vi "Main_Module.vi"(0 "A":dbl, 5 "B":dbl, 11 "Error_In":errorcluster) -> (4 "C":dbl, 15 "Error_Out":errorcluster)   [LabVIEW 2023]
doc: "This is the Main Module that perform the calculator."
uses:
  Controls/Calculator_Operation_Select.ctl
  Controls/Queue_Operation_Select.ctl
  Controls/Calculator_Data.ctl
  Classes/Calculator/Calculator.lvclass
  Controls/State_and_Data.ctl
  Classes/Calculator/Children/Multiplication/Multiplication.lvclass
  D:/Git/Assignments/Assignment-24/Assignment-24_LV23V/Classes/Calculator/Calculator.lvclass
  Classes/Calculator/Children/Division/Division.lvclass
  Classes/Calculator/Children/Addition/Addition.lvclass
  Classes/Calculator/Children/Subtraction/Subtraction.lvclass
panel:
  in  "Operation":T1
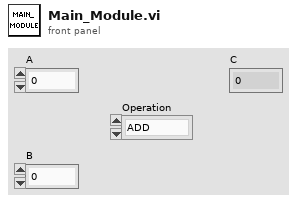
[diagram p1: front panel]
types:
  T1 = typedef "Calculator_Operation_Select.ctl" = enum16{"ADD", "SUB", "MUL", "DIV"}
  T2 = typedef "State_and_Data.ctl" = cluster{"State":string, "Data":variant}
  T3 = typedef "Queue_Operation_Select.ctl" = enum16{"Obtain_Queue", "Enqueue", "Enqueue_First", "Enqueue_N", "Lossy_Enqueue", "Preview", "Queue_Status", "Dequeue", "Flush", "Release_Queue"}
  T4 = typedef "Calculator_Data.ctl" = cluster{"Inputs":dbl[], "Operation":T1, "Parent_Calculator":refnum<class "Calculator.lvclass">[], "C":dbl, "State_and_Data":T2}
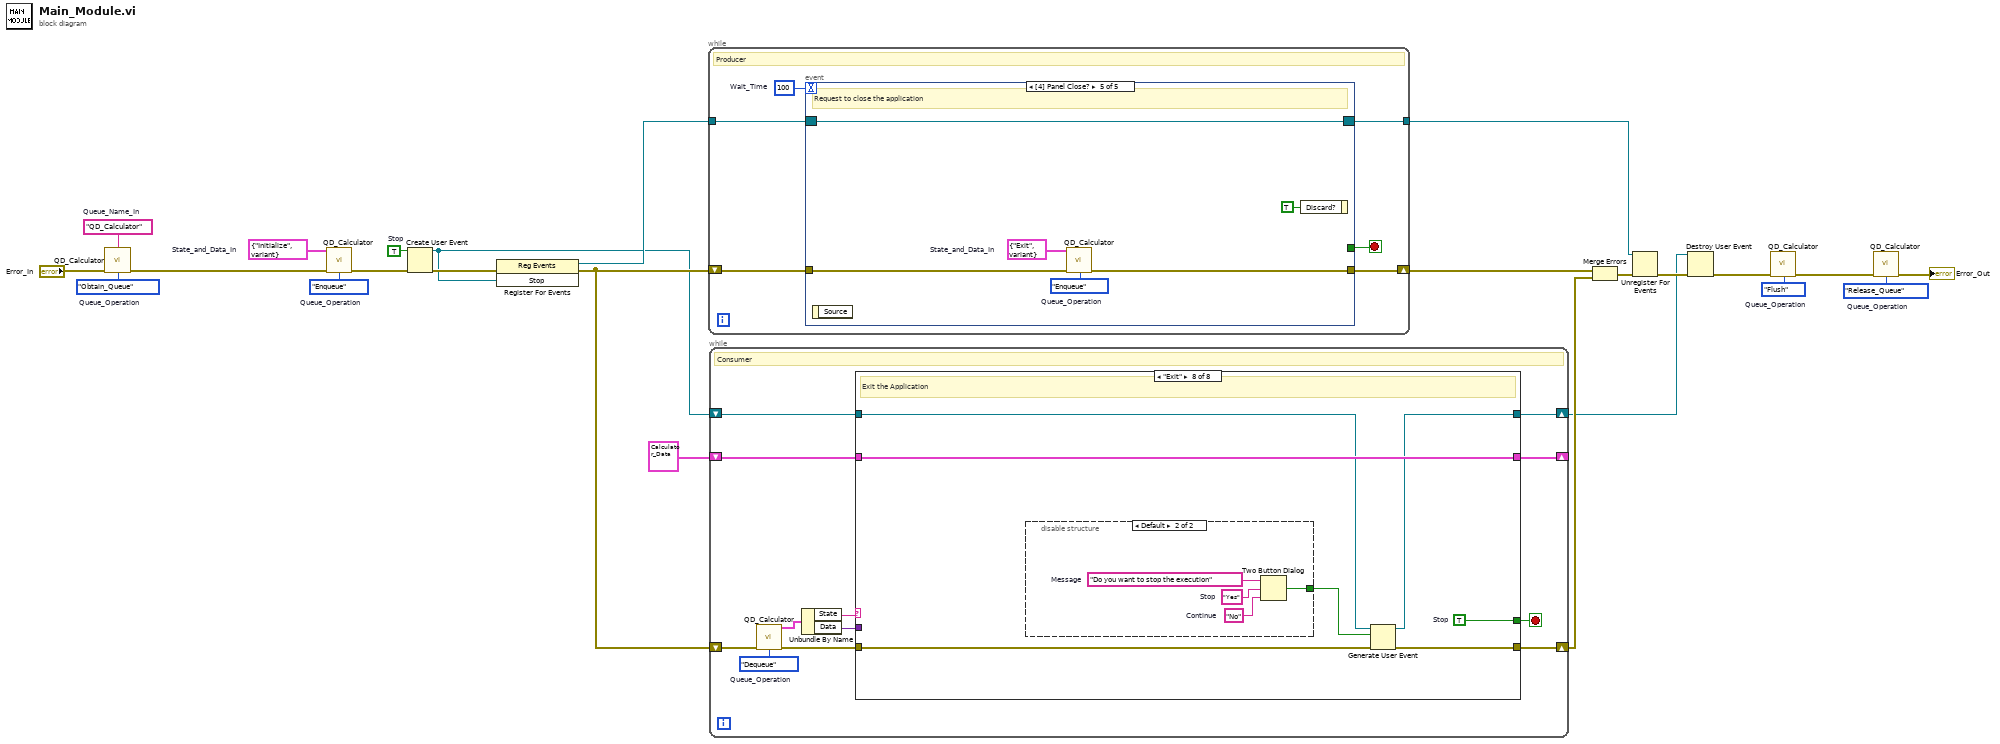
[diagram p0: block diagram]
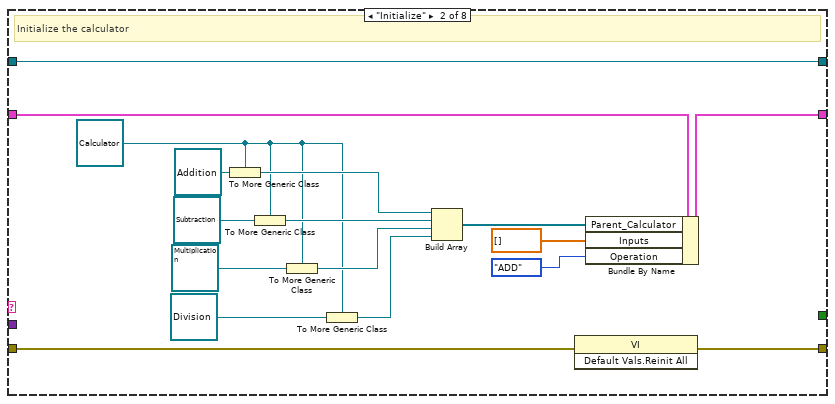
[diagram p3: hidden frame]
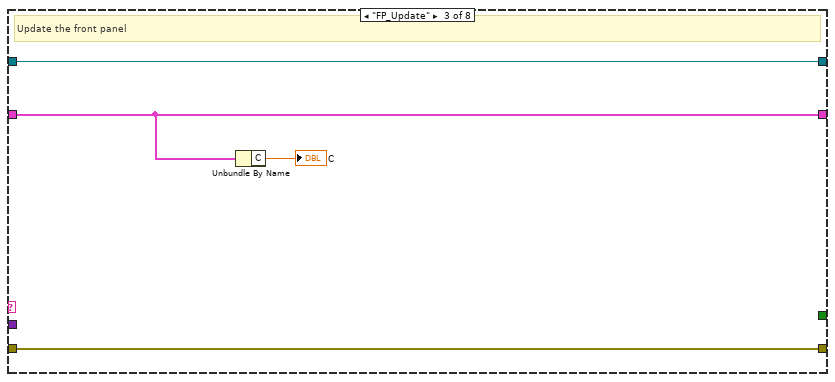
[diagram p4: hidden frame]
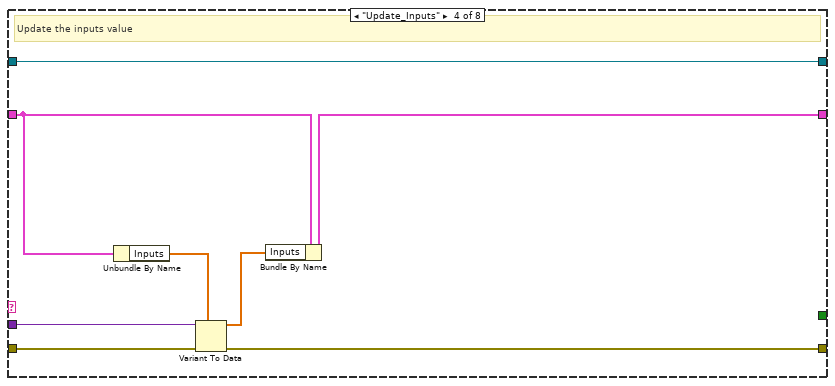
[diagram p5: hidden frame]
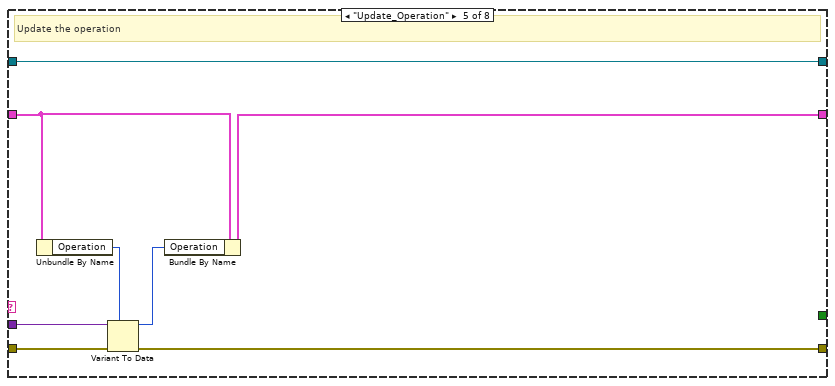
[diagram p6: hidden frame]
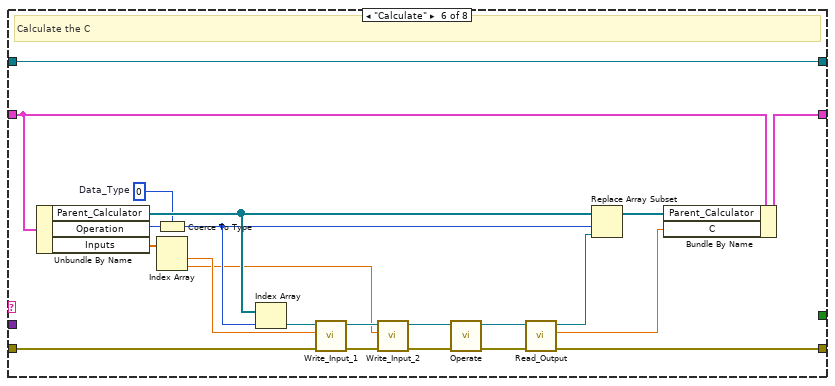
[diagram p7: hidden frame]
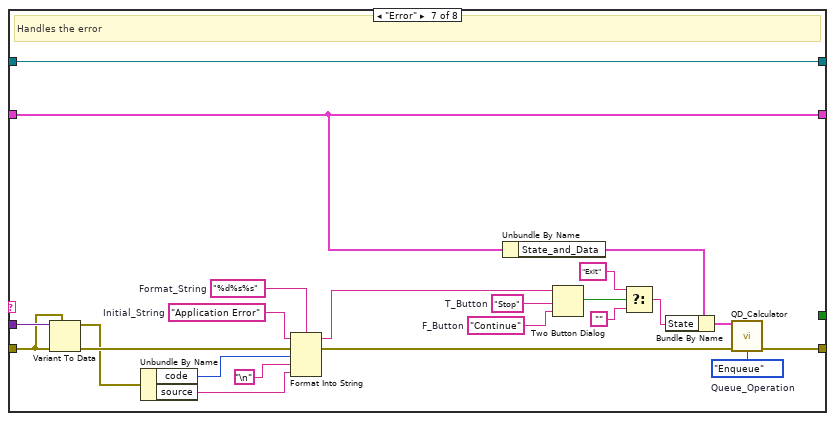
[diagram p8: hidden frame]
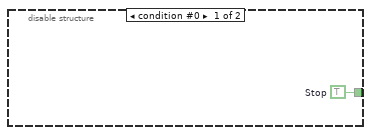
[diagram p9: hidden frame]
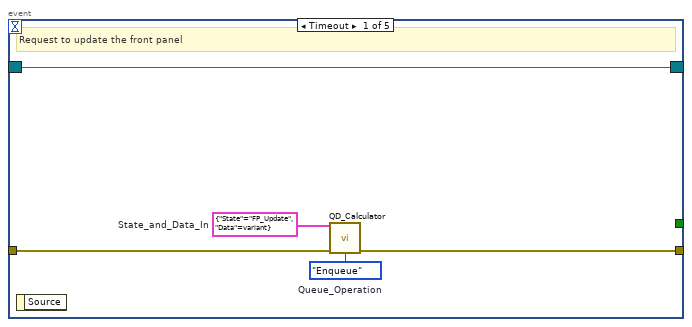
[diagram p10: hidden frame]
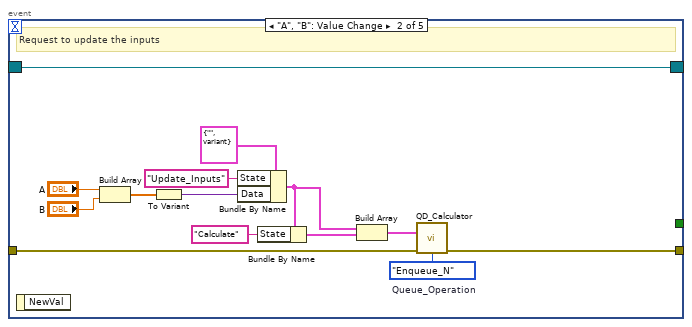
[diagram p11: hidden frame]
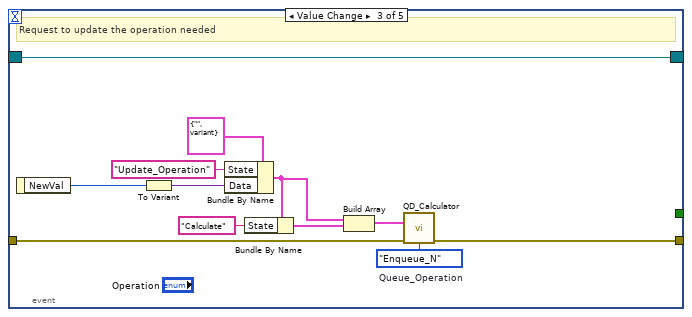
[diagram p12: hidden frame]
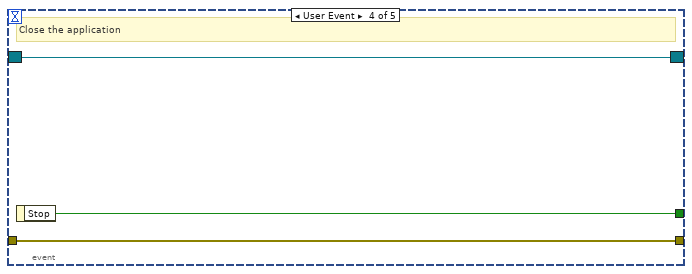
[diagram p13: hidden frame]
diagram:
  w1 = T2 {"State"="Initialize", "Data"=variant}  # State_and_Data_In
  w2 = Queue_Operation_Select."Release_Queue"  # Queue_Operation
  w3 = Queue_Operation_Select."Flush"  # Queue_Operation
  w6 = TRUE  # Stop
  w16 = "QD_Calculator"  # Queue_Name_In
  w17 = Queue_Operation_Select."Enqueue"  # Queue_Operation
  w18 = Queue_Operation_Select."Obtain_Queue"  # Queue_Operation
  n1 = call "QD_Calculator.vi"("Queue_Name_In"=w16, "Error_In"="Error_In", "Queue_Operation"=w18) -> ("Error_Out"=w20:errorcluster)  [unwired: 10 in, 2 out]
  n2 = call "QD_Calculator.vi"("State_and_Data_In"=w1, "Error_In"=w20, "Queue_Operation"=w17) -> ("Error_Out"=w19:errorcluster)  [unwired: 10 in, 2 out]
  n3 = Create User Event(user event datatype=w6, error in=w19) -> (user event=w7:refnum<user-event>, error out=w14:errorcluster)
  n4 = register-events(error in=w14, w7) -> (reference out=w12:refnum<event-registration>, error out=w13:errorcluster)  [unwired: 1 in]
  n5 = while {
    shift-right: [w29] -> w24
    shift-left: w13 -> [w30]
    tunnel: w12 -> [w27]
    tunnel: [w26] -> w10
    stop <- w25 stop-if-true
    w28 = 100  # Wait_Time
    # "Producer"
    n6 = event shown="[4] Panel Close?" {
      selector: w27 -> [w34 w39 w50 w62 w65]
      dyn-events: [w34 w39 w50 w62 w65] -> w26
      timeout: w28 -> [_ _ _ _ _]
      tunnel: w30 -> [w35 w40 w61 w64 w70]
      tunnel: [w33 w41 w60 w64 w69] -> w29
      tunnel: [_ _ _ w63 _] -> w25
      event Timeout {
        w31 = T2 {"State"="FP_Update", "Data"=variant}  # State_and_Data_In
        w32 = Queue_Operation_Select."Enqueue"  # Queue_Operation
        # "Request to update the front panel"
        n7 = event-data() -> ()  [unwired: 1 in, 1 out]
        n8 = call "QD_Calculator.vi"("State_and_Data_In"=w31, "Error_In"=w35, "Queue_Operation"=w32) -> ("Error_Out"=w33:errorcluster)  [unwired: 10 in, 2 out]
      }
      event "A", "B": Value Change {
        w49 = Queue_Operation_Select."Enqueue_N"  # Queue_Operation
        # "Request to update the inputs"
        n9 = event-data() -> ()  [unwired: 1 in, 1 out]
        n10 = Build Array("A", "B") -> (w36:dbl[])
        n11 = To Variant(anything=w36) -> (Variant=w47:variant)
        n12 = Bundle By Name(cluster=T2 {"State"="", "Data"=variant} ("State_and_Data"), "State"="Update_Inputs", "Data"=w47) -> (w45:T2)
        n13 = Bundle By Name(cluster=w45, "State"="Calculate") -> (w44:T2)
        n14 = Build Array(w45, w44) -> (w43:T2[])
        n15 = call "QD_Calculator.vi"("State_and_Data_N_In"=w43, "Error_In"=w40, "Queue_Operation"=w49) -> ("Error_Out"=w41:errorcluster)  [unwired: 10 in, 2 out]
      }
      event Value Change {
        w59 = Queue_Operation_Select."Enqueue_N"  # Queue_Operation
        # "Request to update the operation needed"
        n16 = event-data() -> ("NewVal"=w57:T1)  [unwired: 1 in]
        n17 = To Variant(anything=w57) -> (Variant=w56:variant)
        n18 = Bundle By Name(cluster=T2 {"State"="", "Data"=variant} ("State_and_Data"), "State"="Update_Operation", "Data"=w56) -> (w54:T2)
        n19 = Bundle By Name(cluster=w54, "State"="Calculate") -> (w53:T2)
        n20 = Build Array(w54, w53) -> (w52:T2[])
        n21 = call "QD_Calculator.vi"("State_and_Data_N_In"=w52, "Error_In"=w61, "Queue_Operation"=w59) -> ("Error_Out"=w60:errorcluster)  [unwired: 10 in, 2 out]
      }
      event User Event {
        # "Close the application"
        n22 = event-data() -> ("Stop"=w63:bool)  [unwired: 1 in]
      }
      event Panel Close? {
        w67 = T2 {"State"="Exit", "Data"=variant}  # State_and_Data_In
        w68 = Queue_Operation_Select."Enqueue"  # Queue_Operation
        # "Request to close the application"
        n23 = event-data() -> ()  [unwired: 1 in, 1 out]
        n24 = call "QD_Calculator.vi"("State_and_Data_In"=w67, "Error_In"=w70, "Queue_Operation"=w68) -> ("Error_Out"=w69:errorcluster)  [unwired: 10 in, 2 out]
        n25 = event-data("Discard?"=TRUE) -> ()  [unwired: 1 in, 1 out]
      }
    }
  }
  n26 = while {
    shift-right: [w81] -> w21
    shift-left: w13 -> [w82]
    shift-right: [w75] -> _
    shift-left: T4 {"Inputs"=[], "Operation"=enum."ADD", "Parent_Calculator"=[], "C"=0.0, "State_and_Data"={"State"="", "Data"=variant}} -> [w74]
    shift-right: [w73] -> w8
    shift-left: w7 -> [w72]
    stop <- w71 stop-if-true
    w79 = Queue_Operation_Select."Dequeue"  # Queue_Operation
    # "Consumer"
    n27 = call "QD_Calculator.vi"("Error_In"=w82, "Queue_Operation"=w79) -> ("State_and_Data_Out"=w78:T2, "Error_Out"=w80:errorcluster)  [unwired: 11 in, 1 out]
    n28 = Unbundle By Name(w78) -> ("State"=w77:string, "Data"=w76:variant)
    n29 = case shown="\"Exit\"" w77 {
      tunnel: w80 -> [w85 w102 w106 w114 w122 w143 w150 w174]
      tunnel: [w85 w86 w106 w113 w121 w135 w147 w172] -> w81
      tunnel: w76 -> [_ _ _ w112 w120 _ w151 _]
      tunnel: [w84 w100 w104 w109 w117 w137 w153 w173] -> w75
      tunnel: w74 -> [w84 w101 w104 w110 w118 w144 w153 w173]
      tunnel: [w83 w87 w105 w107 w115 w127 w167 w170] -> w73
      tunnel: w72 -> [w83 w87 w105 w107 w115 w127 w167 w171]
      tunnel: [_ _ _ _ _ _ _ w169] -> w71
      frame Default {
      }
      frame "Initialize" {
        w90 = refnum<class "Calculator.lvclass"> refnum ("Calculator.lvclass")
        # "Initialize the calculator"
        n30 = To More Generic Class(target class=w90, reference=refnum<class "Addition.lvclass"> refnum ("Addition.lvclass")) -> (generic class reference=w94:refnum<class "Calculator.lvclass">)
        n31 = To More Generic Class(target class=w90, reference=refnum<class "Subtraction.lvclass"> refnum ("Subtraction.lvclass")) -> (generic class reference=w93:refnum<class "Calculator.lvclass">)
        n32 = To More Generic Class(target class=w90, reference=refnum<class "Multiplication.lvclass"> refnum ("Multiplication.lvclass")) -> (generic class reference=w92:refnum<class "Calculator.lvclass">)
        n33 = To More Generic Class(target class=w90, reference=refnum<class "Division.lvclass"> refnum ("Division.lvclass")) -> (generic class reference=w91:refnum<class "Calculator.lvclass">)
        n34 = Build Array(w94, w93, w92, w91) -> (w95:refnum<class "Calculator.lvclass">[])
        n35 = invoke class="VI" method="Default Vals.Reinit All"(error in=w102) -> (error out=w86:errorcluster)  [unwired: 2 in, 2 out]
        n36 = Bundle By Name(cluster=w101, "Parent_Calculator"=w95, "Inputs"=dbl[] [] ("A"), "Operation"=Calculator_Operation_Select."ADD") -> (w100:T4)
      }
      frame "FP_Update" {
        # "Update the front panel"
        n37 = Unbundle By Name(w104) -> ("C"=→"C":dbl)
      }
      frame "Update_Inputs" {
        # "Update the inputs value"
        n38 = Unbundle By Name(w110) -> ("Inputs"=w111:dbl[])
        n39 = Variant To Data(error in=w114, type=w111, Variant=w112) -> (data=w108:dbl[], error out=w113:errorcluster)
        n40 = Bundle By Name(cluster=w110, "Inputs"=w108) -> (w109:T4)
      }
      frame "Update_Operation" {
        # "Update the operation"
        n41 = Unbundle By Name(w118) -> ("Operation"=w119:T1)
        n42 = Variant To Data(error in=w122, type=w119, Variant=w120) -> (data=w116:T1, error out=w121:errorcluster)
        n43 = Bundle By Name(cluster=w118, "Operation"=w116) -> (w117:T4)
      }
      frame "Calculate" {
        w128 = 0  # Data_Type
        # "Calculate the C"
        n44 = Unbundle By Name(w144) -> ("Parent_Calculator"=w133:refnum<class "Calculator.lvclass">[], "Operation"=w132:T1, "Inputs"=w125:dbl[])
        n45 = Coerce To Type(0:w132, 1:w128) -> (2:w129:i32)
        n46 = Index Array(array=w125) -> (element #1=w124:dbl, element #2=w123:dbl)  [unwired: 2 in]
        n47 = Index Array(array=w133, index=w129) -> (element=w140:refnum<class "Calculator.lvclass">)
        n48 = call-dynamic "Write_Input_1.vi"("Error_In"=w143, "Input_1"=w124, "Calculator_In"=w140) -> ("Error_Out"=w142:errorcluster, "Calculator_Out"=w126:refnum<class "Calculator.lvclass">)  [unwired: 7 in]
        n49 = call-dynamic "Write_Input_2.vi"("Error_In"=w142, "Input_2"=w123, "Calculator_In"=w126) -> ("Error_Out"=w141:errorcluster, "Calculator_Out"=w139:refnum<class "Calculator.lvclass">)  [unwired: 7 in]
        n50 = call-dynamic "Operate.vi"("Error_In"=w141, "Calculator_In"=w139) -> ("Error_Out"=w136:errorcluster, "Calculator_Out"=w138:refnum<class "Calculator.lvclass">)  [unwired: 8 in]
        n51 = call-dynamic "Read_Output.vi"("Error_In"=w136, "Calculator_In"=w138) -> ("Error_Out"=w135:errorcluster, "Output"=w130:dbl, "Calculator_Out"=w131:refnum<class "Calculator.lvclass">)  [unwired: 7 in]
        n52 = Replace Array Subset(array=w133, new element=w131, index=w129) -> (w134:refnum<class "Calculator.lvclass">[])
        n53 = Bundle By Name(cluster=w144, "Parent_Calculator"=w134, "C"=w130) -> (w137:T4)
      }
      frame "Error" {
        w145 = Queue_Operation_Select."Enqueue"  # Queue_Operation
        w162 = "%d%s%s"  # Format_String
        w163 = "Application Error"  # Initial_String
        w164 = "Stop"  # T_Button
        w165 = "Continue"  # F_Button
        # "Handles the error"
        n54 = Variant To Data(error in=w150, type=w150, Variant=w151) -> (data=w149:errorcluster, error out=w152:errorcluster)
        n55 = Unbundle By Name(w149) -> ("code"=w160:i32, "source"=w159:string)
        n56 = Format Into String(format string=w162, initial string=w163, error in=w152, w160, "\n", w159) -> (resulting string=w166:string, error out=w154:errorcluster)
        n57 = Unbundle By Name(w153) -> ("State_and_Data"=w148:T2)
        n58 = Two Button Dialog(message=w166, 1:w165, 2:w164) -> (T button?=w157:bool)
        n59 = Select(t="Exit" ("State"), s=w157, f="") -> (s? t:f=w155:string)
        n60 = Bundle By Name(cluster=w148, "State"=w155) -> (w146:T2)
        n61 = call "QD_Calculator.vi"("State_and_Data_In"=w146, "Error_In"=w154, "Queue_Operation"=w145) -> ("Error_Out"=w147:errorcluster)  [unwired: 10 in, 2 out]
      }
      frame "Exit" {
        w169 = TRUE  # Stop
        # "Exit the Application"
        n62 = disable-structure shown="Default" {
          disable-tunnel: [w175 w176] -> w168
          frame condition #0 {
            w175 = TRUE  # Stop
          }
          frame condition #1 (active) {
            w177 = "No"  # Continue
            w178 = "Yes"  # Stop
            w179 = "Do you want to stop the execution"  # Message
            n63 = Two Button Dialog(message=w179, 1:w177, 2:w178) -> (T button?=w176:bool)
          }
        }
        n64 = Generate User Event(user event=w171, event data cluster=w168, error in=w174) -> (user event out=w170:refnum<user-event>, error out=w172:errorcluster)  [unwired: 1 in]
      }
    }
  }
  n65 = Merge Errors(w24, w21) -> (w22:errorcluster)
  n66 = Unregister For Events(event registration refnum=w10, error in=w22) -> (error out=w11:errorcluster)
  n67 = Destroy User Event(user event=w8, error in=w11) -> (error out=w9:errorcluster)
  n68 = call "QD_Calculator.vi"("Error_In"=w9, "Queue_Operation"=w3) -> ("Error_Out"=w4:errorcluster)  [unwired: 11 in, 2 out]
  n69 = call "QD_Calculator.vi"("Error_In"=w4, "Queue_Operation"=w2) -> ("Error_Out"=→"Error_Out":errorcluster)  [unwired: 11 in, 2 out]
